vi "startOpenLoopScan.vi"(0 "WaitForUserInputState in":refnum<class "WaitForUserInputState.lvclass">, 5 "model":refnum<class "Model.lvclass">, 7 "Force Setpoint":dbl[unit], 9 "Center Point":dbl[unit], 11 "error in (no error)":errorcluster) -> (4 "WaitForUserInputState out":refnum<class "WaitForUserInputState.lvclass">, 6 "model 2":refnum<class "Model.lvclass">, 15 "error out":errorcluster)   [LabVIEW 2015, in "WaitForUserInputState.lvclass"]
uses:
  WaitForUserInputState.lvclass
  Model/Model/Model.lvclass
  Typedefs/StateSelector.ctl
  Model/Model/Model.lvclass/Model.ctl
  Typedefs/FAMTTypedefs.lvlib
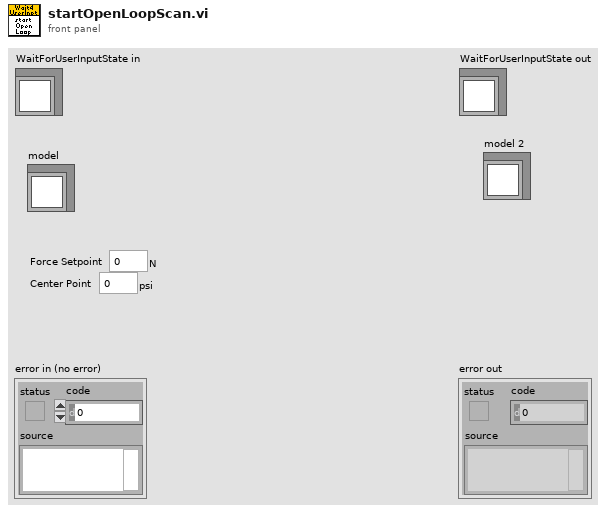
[diagram p1: front panel]
types:
  T1 = typedef "FAMTTypedefs.lvlib/StateSelector.ctl" = enum16{"OfflineState", "FaultState", "StandbyState", "DisabledState", "EnabledState", "WaitForUserInputState", "PerformOpenLoopScanState"}
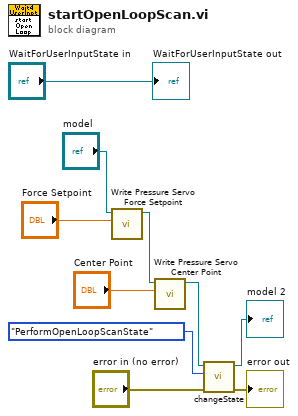
[diagram p0: block diagram]
diagram:
  n1 = call "Write Pressure Servo Force Setpoint.vi"("Pressure Servo Force Setpoint"="Force Setpoint", "Model in"="model") -> ("Model out"=w2:refnum<class "Model.lvclass">)  [unwired: 9 in]
  n2 = call "Write Pressure Servo Center Point.vi"("Pressure Servo Center Point"="Center Point", "Model in"=w2) -> ("Model out"=w3:refnum<class "Model.lvclass">)  [unwired: 9 in]
  n3 = call "changeState.vi"("error in (no error)"="error in (no error)", "State:"=StateSelector."PerformOpenLoopScanState", "Model in"=w3) -> ("error out"=→"error out":errorcluster, "Model out"=→"model 2":refnum<class "Model.lvclass">)  [unwired: 7 in]
  "WaitForUserInputState out" <- "WaitForUserInputState in"
